vi "Host Main.vi"() -> ()   [LabVIEW 2015]
doc: "This application launches and executes the Tag Bus Data framework configuration for the specified target alias. This is a simple example of the framework API functions, but may also be a suitable starting point for a Host UI or Thick Client that is running a local version of the framework."
uses:
  <vilib>/NI/Module Execution Interface/Engine Runtime/Execution States.ctl
  <vilib>/NI/Module Execution Interface/Engine Runtime/Fault.ctl
  <vilib>/NI/Tag Bus Module Framework/runtime/error classification.ctl
  <vilib>/NI/Module Execution Interface/Engine Runtime/Engine Runtime Interface.lvclass
  <vilib>/NI/DCAF/Tag Editor Core/Framework Configuration Classes/target runtime/PL_Target Runtime.lvclass
  <vilib>/NI/Tag Bus Module Framework/FPGA manager/FPGA manager.lvlib
  <vilib>/rvi/interface/nirviOpenFPGA/nirviOpenFPGA.xnode
  <vilib>/userdefined/High Color/nirio_resource_hc.ctl
  <vilib>/NI/Tag Bus Module Framework/FPGA manager/methods.ctl
  <vilib>/NI/Tag Bus Module Framework/runtime/TBM module execution interface.lvclass
panel:
  in  "configuration file path":path
  in  "target alias":string="PC"
  out "engine status":T4(array[cluster])
  in  "stop":bool
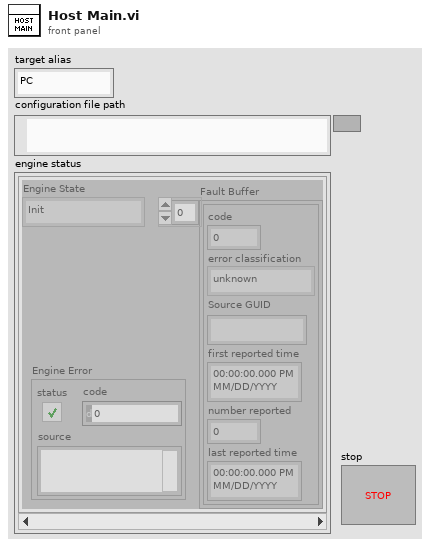
[diagram p1: front panel]
types:
  T1 = typedef "Engine Runtime Interface.lvclass/Execution States.ctl" = enum16{"Init", "Pre-Operational", "Safe-Operational", "Operational", "Stopped"}
  T2 = typedef "Engine Runtime Interface.lvclass/Fault.ctl" = cluster{"code":i32, "error classification":T3, "Source GUID":string, "first reported time":timestamp, "number reported":u32, "last reported time":timestamp}
  T3 = typedef "TBM module execution interface.lvclass/error classification.ctl" = enum16{"unknown", "none", "trivial", "recoverable", "critical"}
  T4 = cluster{"Engine State":T1, "Fault Buffer":T2[], "Engine Error":errorcluster}[]
  T5 = typedef "FPGA manager.lvlib/methods.ctl" = enum16{"initialize bitfile", "cache bitfile", "locate bitfile", "close bitfile", "clear manager"}
  T6 = typedef "nirio_resource_hc.ctl" = tag
  T7 = cluster{"Engine State":T1, "faults":T2[], "Engine Error":errorcluster}
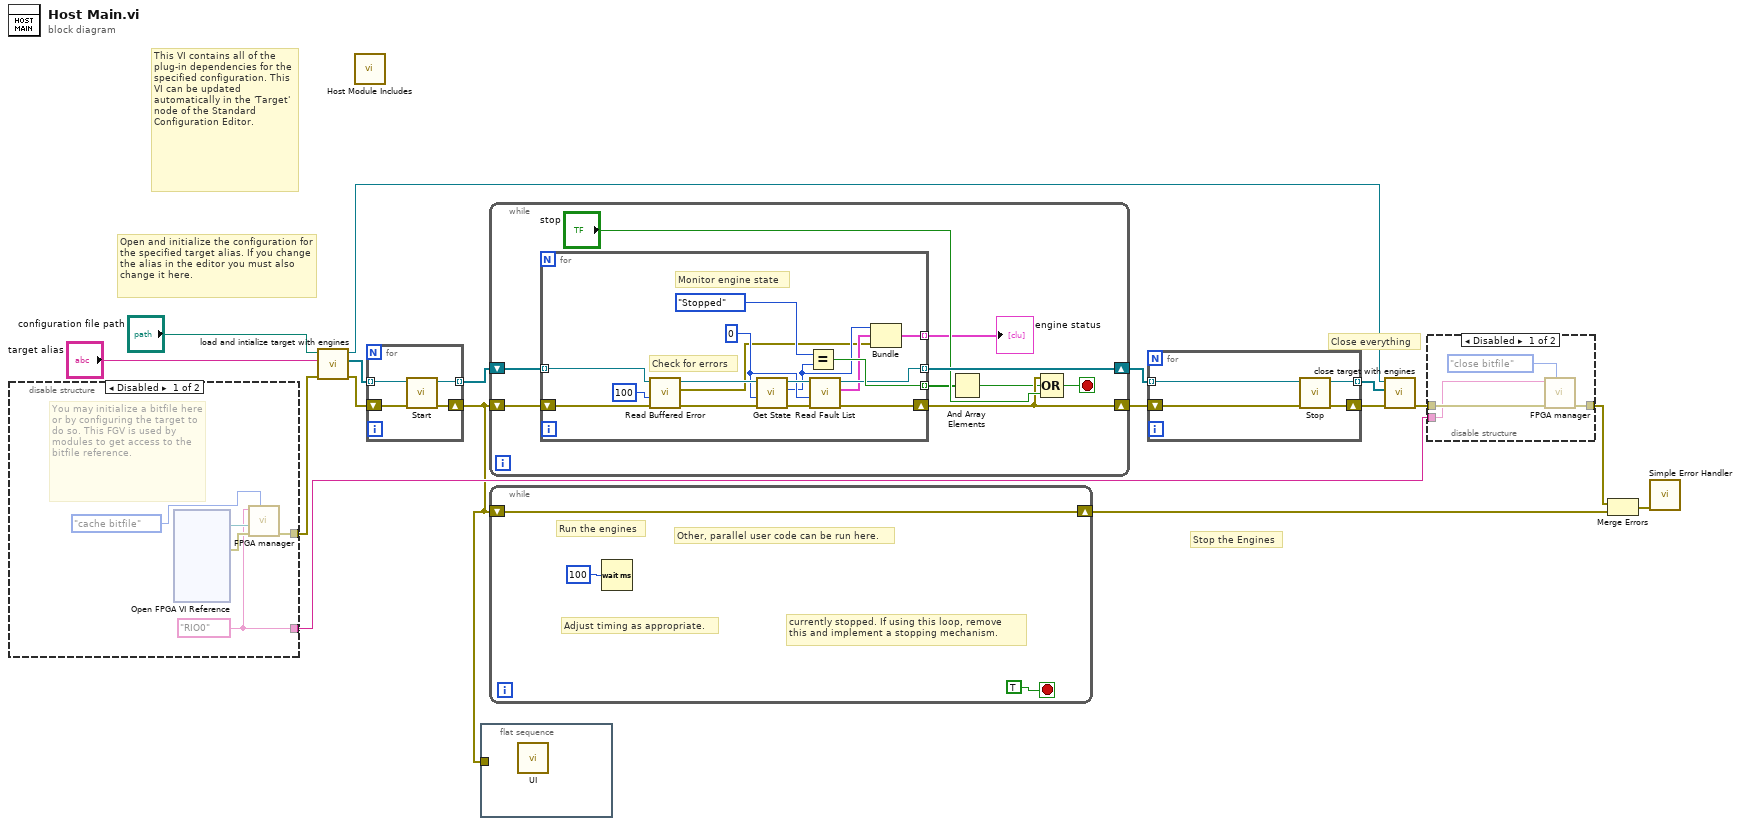
[diagram p0: block diagram]
diagram:
  # "Open and initialize the configuration for the specified target alias. If you change the alias in the editor you must also change it here."
  # "Close everything"
  # "Stop the Engines"
  # "This VI contains all of the plug-in dependencies for the specified configuration. This VI can be updated automatically in the 'Target' node of the Standard Configuration Editor."
  # "Run the engines"
  n1 = disable-structure shown="Disabled" {
    disable-tunnel: [w22 _] -> w7
    disable-tunnel: [w18 _] -> w6
    frame Disabled {
      w18 = T6 "RIO0" ("RIO resource")
      # "You may initialize a bitfile here or by configuring the target to do so. This FGV is used by modules to get access to the bitfile reference."
      n2 = xnode "Open FPGA VI Reference"() -> ("FPGA VI Reference Out"=w20:refnum<k20>, "error out"=w21:errorcluster)  [unwired: 2 in]
      n3 = call <vilib>:"FPGA manager.vi"("action"=methods."cache bitfile", "error in"=w21, "bitfile to cache"=w20, "RIO resource"=w18) -> ("error out"=w22:errorcluster)  [unwired: 5 in, 2 out]
    }
    frame Enabled {
    }
  }
  n4 = call <vilib>:"load and intialize target with engines.vi"("error in"=w7, "target alias"="target alias", "file path"="configuration file path") -> ("error out"=w14:errorcluster, "engine runtime interfaces"=w13:refnum<class "Engine Runtime Interface.lvclass">[], "target runtime"=w10:refnum<class "PL_Target Runtime.lvclass">)  [unwired: 6 in]
  n5 = call "Host Module Includes.vi"() -> ()  [unwired: 12 in]
  n6 = for {
    tunnel: [w26] -> w17 mode=indexing
    tunnel: w13 -> [w23] mode=indexing
    shift-right: [w25] -> w1
    shift-left: w14 -> [w24]
    n7 = call-dynamic "Start.vi"("error in"=w24, "Engine Runtime Interface in"=w23) -> ("error out"=w25:errorcluster, "Engine Runtime Interface out"=w26:refnum<class "Engine Runtime Interface.lvclass">)  [unwired: 8 in]
  }
  n8 = flat-sequence {
    tunnel: w1 -> [_]
    frame #0 {
      n9 = call "UI.vi"() -> ()  [unwired: 12 in]
    }
  }
  n10 = while {
    shift-right: [w33] -> w16
    shift-left: w17 -> [w35]
    shift-right: [w30] -> w15
    shift-left: w1 -> [w34]
    stop <- w31 stop-if-true
    n11 = for {
      tunnel: w35 -> [w51] mode=indexing
      tunnel: [w42] -> w33 mode=indexing
      tunnel: [w46] -> w28 mode=indexing
      shift-right: [w41] -> w30
      shift-left: w34 -> [w50]
      tunnel: [w36] -> w29 mode=indexing
      w40 = 0 ("timeout (-1)")
      # "Monitor engine state"
      # "Check for errors"
      n12 = call-dynamic "Read Buffered Error.vi"("error in"=w50, "timeout in ms (0)"=100, "Engine Runtime Interface in"=w51) -> ("error out"=w48:errorcluster, "Engine Error"=w37:errorcluster, "Engine Runtime Interface out"=w49:refnum<class "Engine Runtime Interface.lvclass">)  [unwired: 6 in]
      n13 = call-dynamic "Get State.vi"("error in"=w48, "timeout (-1)"=w40, "Engine Runtime Interface in"=w49) -> ("error out"=w44:errorcluster, "Engine State"=w39:T1, "Engine Runtime Interface out"=w43:refnum<class "Engine Runtime Interface.lvclass">)  [unwired: 6 in]
      n14 = Equal?(x=Execution_States."Stopped" ("Engine State"), y=w39) -> (x = y?=w46:bool)
      n15 = call-dynamic "Read Fault List.vi"("error in"=w44, "timeout (-1)"=w40, "Engine Runtime Interface in"=w43) -> ("error out"=w41:errorcluster, "faults"=w38:T2[], "Engine Runtime Interface out"=w42:refnum<class "Engine Runtime Interface.lvclass">)  [unwired: 6 in]
      n16 = Bundle("Engine State"=w39, "faults"=w38, "Engine Error"=w37) -> (w36:T7)  [unwired: 1 in]
    }
    "engine status" <- w29
    n17 = And Array Elements(Boolean array=w28) -> (logical AND=w27:bool)
    n18 = Compound Arithmetic op=OR(w30, w27, "stop") -> (w31:bool)
  }
  n19 = while {
    shift-right: [w52] -> w5
    shift-left: w1 -> [w52]
    stop <- TRUE stop-if-true
    # "currently stopped. If using this loop, remove \nthis and implement a stopping mechanism."
    # "Adjust timing as appropriate."
    # "Other, parallel user code can be run here."
    n20 = Wait (ms)(milliseconds to wait=u32 100) -> ()  [unwired: 1 out]
  }
  n21 = for {
    tunnel: w16 -> [w58] mode=indexing
    shift-right: [w55] -> w9
    shift-left: w15 -> [w57]
    tunnel: [w56] -> w11 mode=indexing
    n22 = call-dynamic "Stop.vi"("error in"=w57, "Engine Runtime Interface in"=w58) -> ("error out"=w55:errorcluster, "Engine Runtime Interface out"=w56:refnum<class "Engine Runtime Interface.lvclass">)  [unwired: 8 in]
  }
  n23 = call <vilib>:"close target with engines.vi"("error in"=w9, "Engine Runtime Interfaces"=w11, "Target Runtime"=w10) -> ("error out"=w4:errorcluster)  [unwired: 8 in]
  n24 = disable-structure shown="Disabled" {
    disable-tunnel: [w61 w63] -> w3
    disable-tunnel: w4 -> [w62 w63]
    disable-tunnel: w6 -> [w59 _]
    frame Disabled {
      n25 = call <vilib>:"FPGA manager.vi"("action"=methods."close bitfile", "error in"=w62, "RIO resource"=w59) -> ("error out"=w61:errorcluster)  [unwired: 6 in, 2 out]
    }
    frame Enabled {
    }
  }
  n26 = Merge Errors(w3, w5) -> (w2:errorcluster)
  n27 = call <vilib>:"Simple Error Handler.vi"("error in (no error)"=w2) -> ()  [unwired: 4 in, 5 out]
